vi "Auto_calibrate.vi"(3 "Mode":T4, 5 "Traverse line":T5 {"Row Duration (mins)" format="%#.1f"; "Row No" min=0; "Trace Gas Concentration (%)" min=0.0 format="%#.2f"; "Emission Rate (l/min)" format="%#.2f"; "Tunnel Speed" format="%#.2f"; "Start X" format="%#.2f"; "Start Y" format="%#.2f"; "Start Z" format="%#.2f"; "End X" format="%#.2f"; "End Y" format="%#.2f"; "End Z" format="%#.2f"; "Averaging time (min)" min=0.0 format="%#.2f"}) -> (0 "Error Messages":string, 1 "Status":T2, 2 "Traverse Out":T5 {"Row Duration (mins)" format="%#.1f"; "Row No" min=0; "Trace Gas Concentration (%)" min=0.0 format="%#.2f"; "Emission Rate (l/min)" format="%#.2f"; "Tunnel Speed" format="%#.2f"; "Start X" format="%#.2f"; "Start Y" format="%#.2f"; "Start Z" format="%#.2f"; "End X" format="%#.2f"; "End Y" format="%#.2f"; "End Z" format="%#.2f"; "Averaging time (min)" min=0.0 format="%#.2f"})   [LabVIEW 2012]
uses:
  Gen Trav/Traverse_cluster.ctl
  Gen Trav/Spacing.ctl
  Controls/Multi_run_mode.ctl
  Controls/User_Specific_mode.ctl
  Controls/Auto_Calib_Type.ctl
  Gen Trav/Multi_Run_Status.ctl
  Controls/Auto_Calib_Case.ctl
  File/Setup_Filetype.ctl
  Calibration/Calib_mode.ctl
  Controls/Setup.ctl
  Controls/Post_Process.ctl
  Controls/Save_Data.ctl
  Controls/App_Global.ctl
  Globals/Meas_global.vi
  Globals/Calib_global.vi
  Globals/Trav_pos_global.vi
  <vilib>/Analysis/baseanly.llb/Mean (DBL).vi
  Globals/Extra_Commands_Global.vi
  <vilib>/Analysis/NI_AALBase.lvlib
panel:
  out "Minimum St Dev":dbl[](array[numeric])
  out "Time FFID valve moved":dbl
  out "Wait factor":dbl
  out "Establishment time":string
  out "Orig Calib file string":string
  out "Concentrations":dbl[](array[numeric])
  out "FFID St Dev":dbl[][](array[numeric]) format="%.2f"
  in  "Clear Calib History":bool
  out "Coefficients":dbl[][](array[numeric]) format="%.2f"
  out "Currently in Case":T1
  out "Valve position":dbl format="%.2f"
  out "Currently On":i32
  out "Values":dbl[][](array[numeric]) format="%.2f"
  out "FF Indexes":i16[](array[numeric])
  out "Ch No's":i16[](array[numeric])
  out "No of Calib Points":i32
  out "Root Name":string[](array[string])
  out "Calibration varying":T3
  in  "stop":bool
  out "New Calib Filenames":path[](array[path])
  # "Specific Argument Options\n      Tunnel Speed;1;2;3;4\nOR  Traverse Position\nOR   Concentration"
  # "X           Y            Z"
  # "Start"
  # "End"
  # "X           Y            Z"
  # "Start"
  # "End"
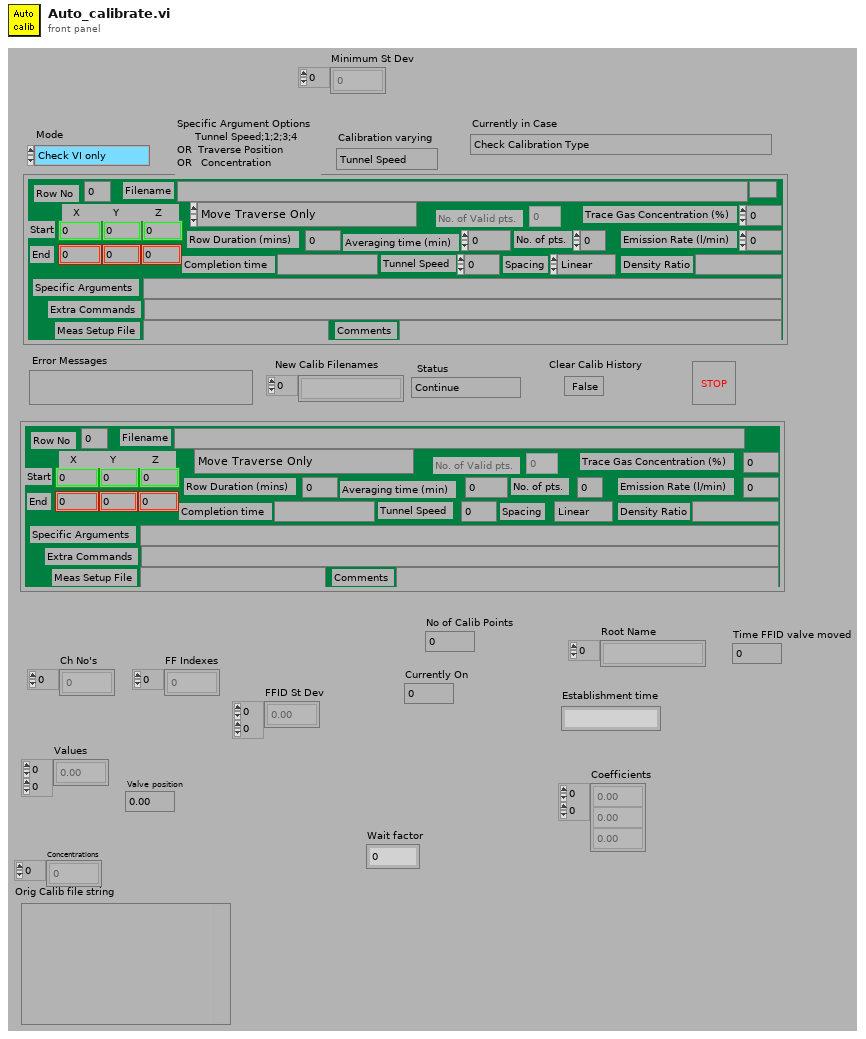
[diagram p1: front panel]
types:
  T1 = typedef "Auto_Calib_Case.ctl" = enum16{"Check Calibration Type", "Check if Original Calib file is Valid", "Get sampling rate etc. from meas setup file", "Setup Calibration Program", "Get Channel Numbers", "Check use latest selected on Mesurement setup files", "Create New Calib Filenames", "Setup Calibration Values in 2D array", "Create Measurement Setup File (Concentration Only)", "Are There Enough Calibration Points", "Set Measurement Conditions", "Measure Calibration Point", "Do Another Calibration Point?", "Skip Next Frame?", "Insert New calibration Filenames into Measurement Setup file", "Warn if FFID calibration is very non linear", "Warn if FFID variance is high", "Insert Bkgnd Variance into calib file", "Warn if FFID voltages are too low", "Warn if Current Calibration fit is poor", "Warn if Calibration Coefficients have significantly altered", "End"}
  T2 = typedef "Multi_Run_Status.ctl" = enum16{"Continue", "Jump to Next Point", "Jump to Next Row", "Jump To Fall Back", "Terminate Run"}
  T3 = typedef "Auto_Calib_Type.ctl" = enum16{"Tunnel Speed", "Traverse Position", "Concentration"}
  T4 = typedef "User_Specific_mode.ctl" = enum16{"Check VI only", "Run VI"}
  T5 = typedef "Traverse_cluster.ctl" = cluster{"Start X":dbl, "Start Y":dbl, "Start Z":dbl, "End X":dbl, "End Y":dbl, "End Z":dbl, "No. of pts.":i32, "Spacing":T6, "Filename":path, "Tunnel Speed":dbl, "Averaging time (min)":dbl, "Extra Commands":string, "Specific Arguments":string, "Emission Rate (l/min)":dbl, "Trace Gas Concentration (%)":dbl, "Density Ratio":string, "Comments":string, "Row No":i32, "Row Type Selector":T7, "Completion time":string, "Row Duration (mins)":dbl, "No. of Valid pts.":i32, "Meas Setup File":string}
  T6 = typedef "Spacing.ctl" = enum16{"Linear", "Log", "Gauss", "Specified", "N/A"}
  T7 = typedef "Multi_run_mode.ctl" = enum16{"Move Traverse Only", "Set Tunnel Speed Only", "Set Source Only", "Set Measurement Conditions", "Single Measurement", "Vertical Profile", "Lateral Profile", "Longitudinal Profile", "Explore Volume", "Multi-Axis Profile", "Auto Calibrate", "Meas Fast FID Bkgnd", "Check Beam Power", "Scanning Valve Measurement", "Run VI Named:", "Set ADAM Ch", "Wait (minutes)", "Send Message", "Synchronize With:", "Fall Back to this Row", "Turn Off Row Repeating", "Blank Row", "Traverse 3D Volume"}
  T8 = typedef "Setup_Filetype.ctl" = enum16{"Measurement Setups", "Calibration Setups", "General", "Results File Plotter Setups", "Speed Calib Tweaks"}
  T9 = typedef "Calib_mode.ctl" = enum16{"Show Setup", "Take a New Calibration Point", "Refit Curve", "Setup Front Panel"}
  T10 = typedef "Save_Data.ctl" = enum16{"Save No Data", "Save Data"}
  T11 = typedef "Post_Process.ctl" = enum16{"Take New Data", "Post Process Raw Data File"}
  T12 = typedef "Setup.ctl" = enum16{"Run Program", "Show Setup", "Save Current Setup", "Setup Front Panel"}
  T13 = typedef "App_Global.ctl" = enum16{"Read Global", "Write to Global", "Initialise Array"}
  T14 = typedef "Cal_Inst_type.ctl" = enum16{"Propeller anemometer", "Pressure Transducer", "Hot wire", "Cross wire velocity", "Cross wire angle", "Generic Linear", "Generic Polynomial", "Generic BackPoly", "Fast FID", "Thermocouple", "Cold wire", "Pulsed Wire"}
  T15 = typedef "Ref_Inst_type.ctl" = enum16{"Propellor anemometer", "Pressure Transducer", "Raw voltage", "Pitot-static tube", "Preston tube", "Generic Linear", "Generic Polynomial", "Thermocouple", "LDA", "Enter Value", "ADAM Channel"}
  T16 = cluster{"2nd Ref type":T15, "2nd inst present":bool}
  T17 = cluster{"high limit (10V)":sgl, "low limit (-10V)":sgl, "Ch No":i16, "Var name":string}[]
  T18 = cluster{"high limit (10V)":sgl, "low limit (-10V)":sgl, "Ch No":i16, "Var name":string}
  T19 = typedef "Inst_type.ctl" = enum16{"Propeller anemometer", "Raw voltage", "Pressure Transducer", "Pitot-static tube", "Preston tube", "Hot wire", "Cross wire 1", "Cross wire 2", "Generic Linear", "Generic Polynomial", "Generic BackPoly", "Fast FID", "Thermocouple", "Cold wire", "Pulsed Wire", "LDA Vel", "LDA Tran time", "LDA Arr time"}
  T20 = cluster{"high limit (10V)":sgl, "low limit (-10V)":sgl, "Ch No":i16, "Calib filename":path, "Inst type":T19, "Symbol":string, "Move channel":bool, "Use Latest":bool, "D":dbl, "Ch Name":string}[]
  T21 = typedef "Status_Cluster.ctl" = cluster{"Status":T2, "Error Type":string, "Error Description":string}
  T22 = typedef "Valco_valve_ph.ctl" = u16
  T23 = typedef "Time_Trace_Cluster.ctl" = cluster{"Weighting":dbl[], "Time (s)":dbl[], "Voltage":dbl[], "Eng Values":dbl[]}
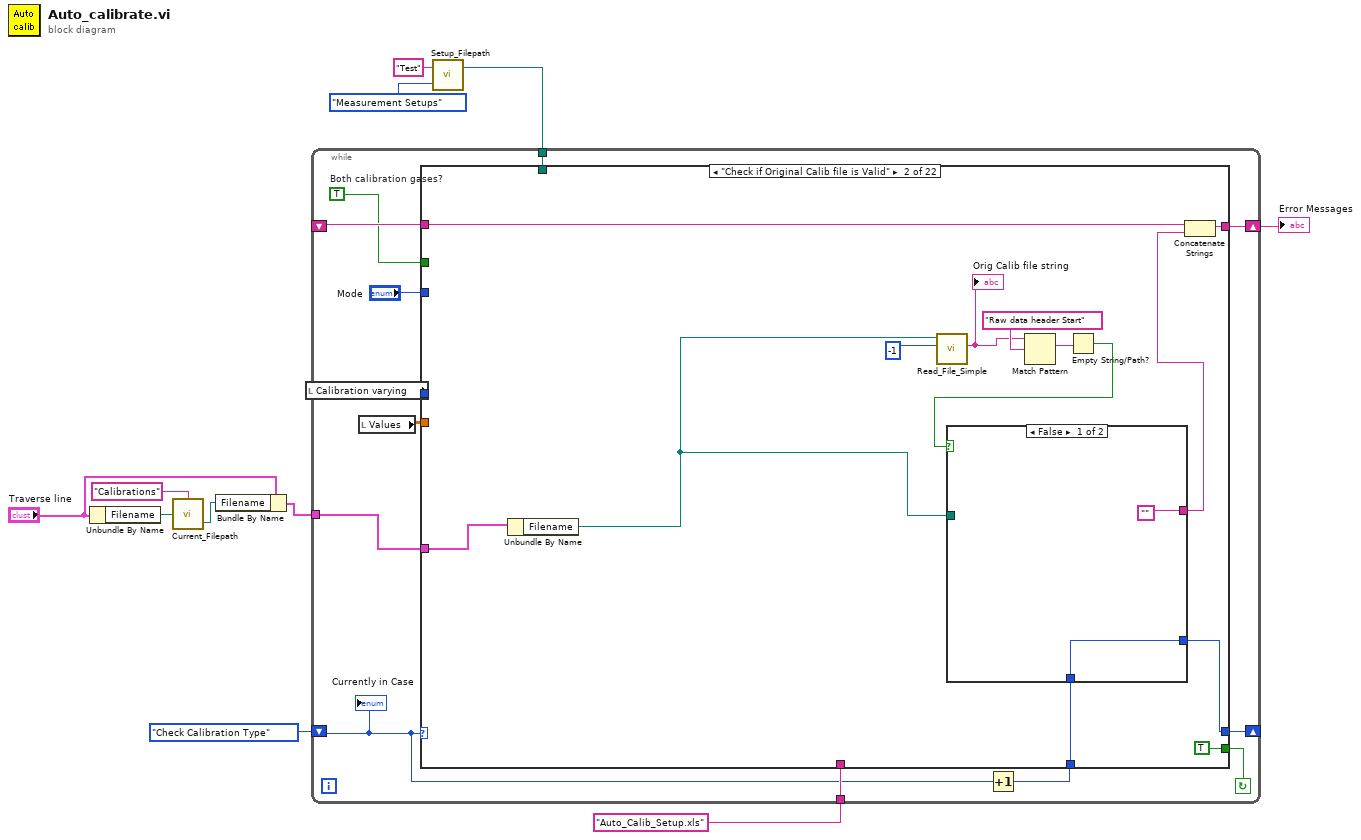
[diagram p0: block diagram]
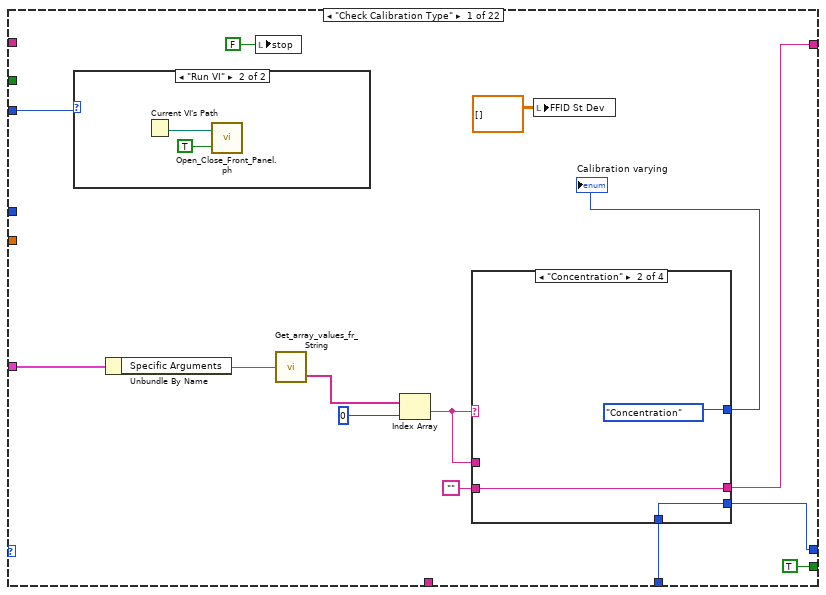
[diagram p2: hidden frame]
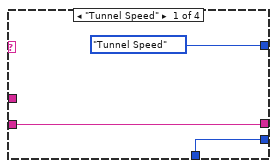
[diagram p4: hidden frame]
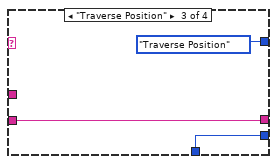
[diagram p5: hidden frame]
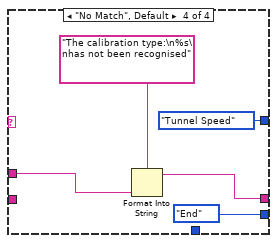
[diagram p6: hidden frame]
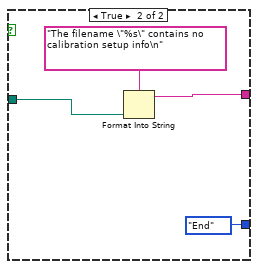
[diagram p7: hidden frame]
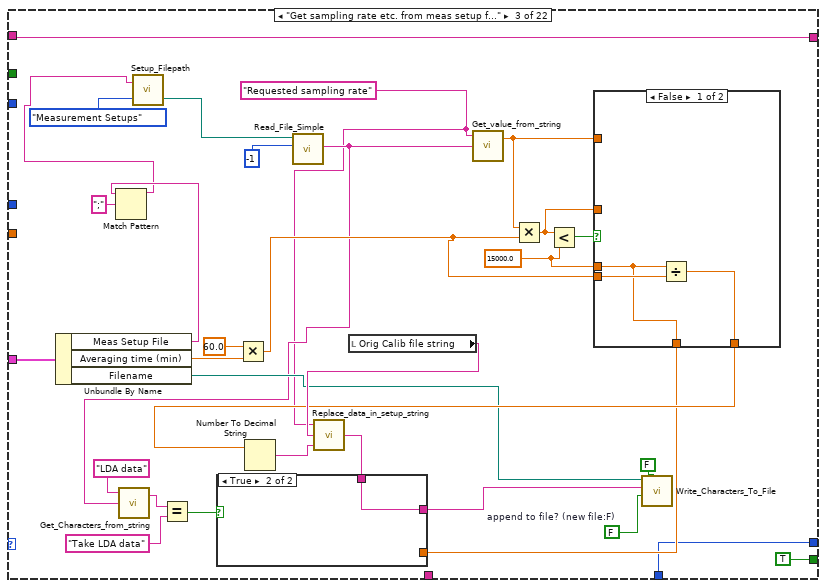
[diagram p8: hidden frame]
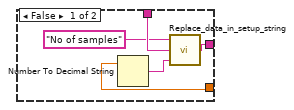
[diagram p9: hidden frame]
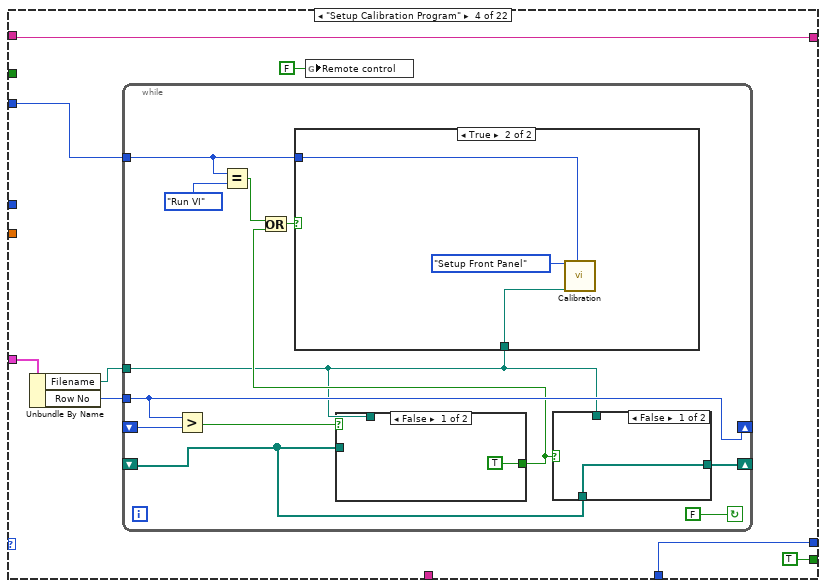
[diagram p11: hidden frame]
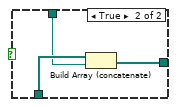
[diagram p12: hidden frame]
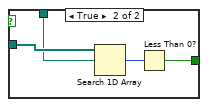
[diagram p14: hidden frame]
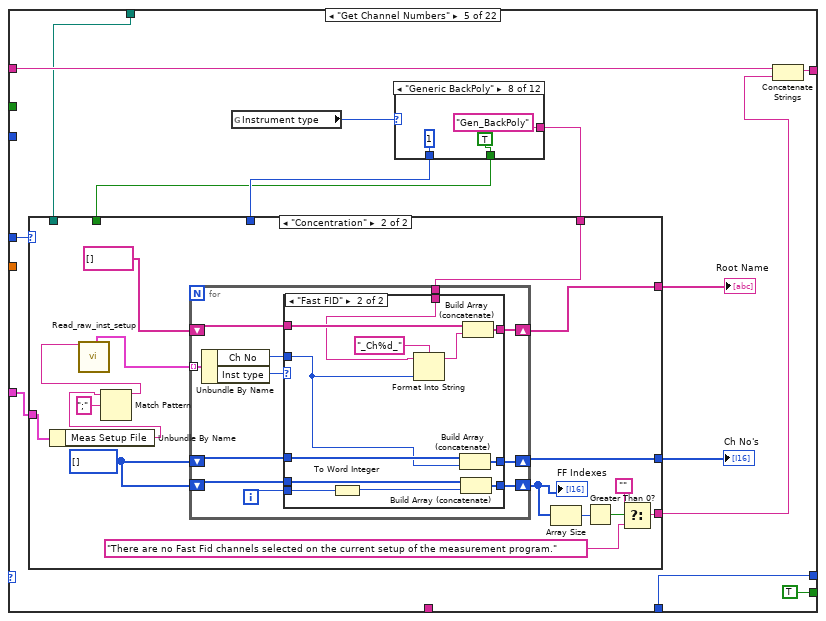
[diagram p15: hidden frame]
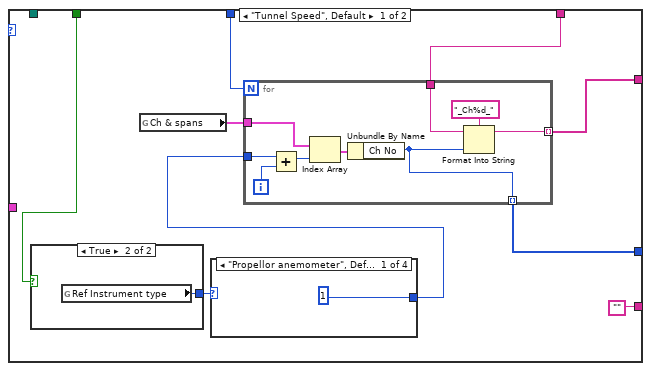
[diagram p16: hidden frame]
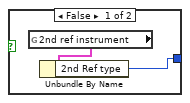
[diagram p17: hidden frame]
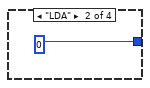
[diagram p18: hidden frame]
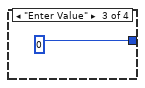
[diagram p19: hidden frame]
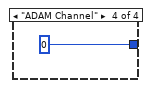
[diagram p20: hidden frame]
diagram:
  n1 = Unbundle By Name("Traverse line") -> ("Filename"=w4:path)
  n2 = call "Current_Filepath.vi"("Filename in"=w4, "Data Type"="Calibrations") -> ("Filename Out"=w3:path)  [unwired: 1 out]
  n3 = Bundle By Name(cluster="Traverse line", "Filename"=w3) -> (w1:T5)
  n4 = call "Setup_Filepath.vi"("Setup File Type"=Setup_Filetype."Measurement Setups", "Filename in"="Test") -> ("Directory"=w6:path)  [unwired: 1 out]
  n5 = while {
    shift-left: _ -> [w17]
    shift-right: [w18] -> w10
    shift-left: Auto_Calib_Case."Check Calibration Type" ("Currently in Case") -> [w16]
    shift-right: [w15] -> _
    tunnel: "Auto_Calib_Setup.xls" -> [w24]
    tunnel: w6 -> [w13]
    tunnel: w1 -> [w12]
    stop <- w21 continue-if-true
    w14 = TRUE  # Both calibration gases?
    n6 = local read "Calibration varying"() -> (w20:T3)
    n7 = local read "Values"() -> (w19:dbl[][])
    n8 = Increment(x=w16) -> (x+1=w22:T1)
    n9 = case shown="\"Check if Original Calib file is Valid\"" w16 {
      tunnel: w12 -> [w38 w67 w105 w120 w151 _ w319 w374 w407 _ w560 _ _ _ _ _ _ _ _ _ w977 w1008]
      tunnel: "Mode" -> [w29 _ _ w121 _ _ w326 _ w408 _ w555 _ w721 _ _ _ _ _ _ _ _ w1009]
      tunnel: w24 -> [_ _ _ _ _ _ _ _ w412 _ _ w632 _ _ _ _ _ _ _ _ _ _]
      tunnel: [w27 w57 w87 w123 w154 w270 w323 w365 w410 w523 w548 w631 w722 w748 w760 w779 w817 w882 w900 w956 w1000 w1013] -> w15
      tunnel: w22 -> [w28 w56 w87 w123 w154 w270 w323 w366 w410 w522 w542 w631 _ w747 w759 w779 w817 w882 w900 w956 w1000 w1013]
      tunnel: [TRUE TRUE TRUE TRUE TRUE TRUE TRUE TRUE w406 TRUE TRUE TRUE TRUE TRUE TRUE TRUE TRUE TRUE TRUE TRUE TRUE FALSE] -> w21
      tunnel: w20 -> [_ _ _ _ w158 _ w322 w372 _ _ w546 w633 w720 w746 w762 _ _ _ _ _ _ w1010]
      tunnel: w19 -> [_ _ _ _ _ _ _ _ w405 w532 w559 _ _ _ _ _ w824 _ w906 _ _ _]
      tunnel: [w31 w59 w85 w124 w155 w271 w336 w369 w411 w526 w543 w629 w719 w751 w766 w788 w831 w878 w907 w945 w993 w1012] -> w18
      tunnel: w17 -> [_ w61 w85 w124 w157 w271 w336 w368 w411 w527 w543 w629 w719 w751 w766 w788 w831 w878 w907 w945 w993 w1012]
      tunnel: w14 -> [_ _ _ _ _ _ _ w367 _ _ _ _ _ _ _ _ _ _ _ _ _ w1007]
      tunnel: w13 -> [_ _ _ _ w150 w273 _ _ w409 _ _ _ _ _ _ _ _ _ _ _ _ _]
      frame "Check Calibration Type" {
        n10 = case shown="\"Run VI\"" w29 {
          frame "Check VI only" {
          }
          frame "Run VI" {
            n11 = Current VI's Path() -> (path=w39:path)
            n12 = call "Open_Close_Front_Panel.ph.vi"("Front Panel Window:Open"=TRUE, "VI path"=w39) -> ()  [unwired: 2 out]
          }
        }
        n13 = Unbundle By Name(w38) -> ("Specific Arguments"=w37:string)
        n14 = local write "stop"(FALSE) -> ()
        n15 = call "Get_array_values_fr_String.vi"("String Value"=w37) -> ("String array"=w36:string[])  [unwired: 1 out]
        n16 = Index Array(array=w36, index=0 ("Index")) -> (element=w34:string)
        n17 = case shown="\"Concentration\"" w34 {
          tunnel: [Auto_Calib_Type."Tunnel Speed" ("Calibration varying") Auto_Calib_Type."Concentration" ("Calibration varying") Auto_Calib_Type."Traverse Position" ("Calibration varying") Auto_Calib_Type."Tunnel Speed" ("Calibration varying")] -> w32
          tunnel: w34 -> [_ _ _ w53]
          tunnel: [w42 w45 w48 w51] -> w31
          tunnel: "" -> [w42 w45 w48 _]
          tunnel: w28 -> [w41 w44 w47 _]
          tunnel: [w41 w44 w47 Auto_Calib_Case."End" ("Currently in Case")] -> w27
          frame "Tunnel Speed" {
          }
          frame "Concentration" {
            (unwired) ""
          }
          frame "Traverse Position" {
          }
          frame "No Match", Default {
            n18 = Format Into String(format string="The calibration type:\n%s\nhas not been recognised" ("Format String"), w53) -> (resulting string=w51:string)  [unwired: 2 in, 1 out]
          }
        }
        "Calibration varying" <- w32
        n19 = local write "FFID St Dev"(dbl[][] [] ("FFID Variance")) -> ()
      }
      frame "Check if Original Calib file is Valid" {
        n20 = Unbundle By Name(w67) -> ("Filename"=w55:path)
        n21 = call "Read_File_Simple.vi"("Filename"=w55, "number of characters (all:-1)"=-1) -> ("string"=w64:string)  [unwired: 1 in, 7 out]
        "Orig Calib file string" <- w64
        n22 = Match Pattern(string=w64, regular expression="Raw data header Start") -> (match substring=w63:string)  [unwired: 4 out]
        n23 = Empty String/Path?(string/path=w63) -> (empty?=w62:bool)
        n24 = case shown="False" w62 {
          tunnel: w55 -> [_ w73]
          tunnel: ["" w71] -> w60
          tunnel: [w68 Auto_Calib_Case."End" ("Currently in Case")] -> w57
          tunnel: w56 -> [w68 _]
          frame False {
          }
          frame True {
            n25 = Format Into String(format string="The filename \"%s\" contains no calibration setup info\n" ("Format String"), w73) -> (resulting string=w71:string)  [unwired: 2 in, 1 out]
          }
        }
        n26 = Concatenate Strings(w61, w60) -> (w59:string)
      }
      frame "Get sampling rate etc. from meas setup file" {
        w88 = FALSE  # append to file? (new file:F)
        w77 = "Requested sampling rate"
        w95 = 15000.0 ("y")
        n27 = Unbundle By Name(w105) -> ("Meas Setup File"=w83:string, "Averaging time (min)"=w103:dbl, "Filename"=w90:path)
        n28 = Match Pattern(string=w83, regular expression=";") -> (before substring=w75:string)  [unwired: 4 out]
        n29 = call "Setup_Filepath.vi"("Setup File Type"=Setup_Filetype."Measurement Setups", "Filename in"=w75) -> ("Filename Out"=w74:path)  [unwired: 1 out]
        n30 = Multiply(x=60.0, y=w103) -> (x*y=w94:dbl)
        n31 = call "Read_File_Simple.vi"("Filename"=w74, "number of characters (all:-1)"=-1) -> ("string"=w82:string)  [unwired: 1 in, 7 out]
        n32 = call "Get_Characters_from_string.vi"("Input string"=w82, "Variable name"="LDA data") -> ("Value"=w80:string)  [unwired: 1 in, 1 out]
        n33 = Equal?(x=w80, y="Take LDA data") -> (x = y?=w78:bool)
        n34 = local read "Orig Calib file string"() -> (w99:string)
        n35 = call "Get_value_from_string.vi"("Input string"=w82, "Variable name"=w77) -> ("Value"=w98:dbl)  [unwired: 1 in, 1 out]
        n36 = Multiply(x=w98, y=w94) -> (x*y=w93:dbl)
        n37 = Less?(x=w93, y=w95) -> (x < y?=w101:bool)
        n38 = case shown="False" w101 {
          tunnel: w98 -> [_ w116]
          tunnel: [w113 w116] -> w97
          tunnel: w95 -> [w112 _]
          tunnel: w94 -> [w114 _]
          tunnel: [w112 w115] -> w91
          tunnel: w93 -> [_ w115]
          frame False {
            n39 = Divide(x=w112, y=w114) -> (x/y=w113:dbl)
          }
          frame True {
          }
        }
        n40 = Number To Decimal String(number=w97) -> (decimal integer string=w96:string)  [unwired: 1 out]
        n41 = call "Replace_data_in_setup_string.vi"("New data string"=w96, "Input string"=w99, "Variable name"=w77) -> ("Appended string"=w92:string)
        n42 = case shown="True" w78 {
          tunnel: w92 -> [w110 w111]
          tunnel: w91 -> [w107 _]
          tunnel: [w106 w111] -> w89
          frame False {
            n43 = Number To Decimal String(number=w107) -> (decimal integer string=w108:string)  [unwired: 1 out]
            n44 = call "Replace_data_in_setup_string.vi"("New data string"=w108, "Input string"=w110, "Variable name"="No of samples") -> ("Appended string"=w106:string)
          }
          frame True {
          }
        }
        n45 = call "Write_Characters_To_File.vi"("file path (dialog if empty)"=w90, "advisory dialog? (display:T)"=FALSE, "character string"=w89, "append to file? (new file:F)"=w88) -> ()  [unwired: 1 in, 4 out]
      }
      frame "Setup Calibration Program" {
        n46 = Unbundle By Name(w120) -> ("Filename"=w117:path, "Row No"=w119:i32)
        n47 = while {
          shift-left: _ -> [w128]
          shift-right: [w127] -> _
          tunnel: w119 -> [w135]
          shift-left: _ -> [w136]
          shift-right: [w135] -> _
          tunnel: w121 -> [w133]
          tunnel: w117 -> [w125]
          stop <- FALSE continue-if-true
          n48 = Greater?(x=w135, y=w136) -> (0:w134:bool)
          n49 = Equal?(x=w133, y=User_Specific_mode."Run VI" ("Mode")) -> (x = y?=w131:bool)
          n50 = case shown="False" w134 {
            tunnel: w128 -> [_ w148]
            tunnel: w125 -> [_ w147]
            tunnel: [TRUE w145] -> w129
            frame False {
            }
            frame True {
              n51 = Search 1D Array(1D array=w148, element=w147) -> (index of element=w146:i32)  [unwired: 1 out]
              n52 = Less Than 0?(x=w146) -> (x < 0?=w145:bool)
            }
          }
          n53 = Or(x=w131, y=w129) -> (x .or. y?=w130:bool)
          n54 = case shown="True" w130 {
            tunnel: w133 -> [_ w143]
            tunnel: w125 -> [_ w142]
            frame False {
            }
            frame True {
              n55 = call "Calibration.vi"("Mode"=Calib_mode."Setup Front Panel", "Calib file"=w142, "Simulate/Run"=w143) -> ()  [unwired: 17 out]
            }
          }
          n56 = case shown="False" w129 {
            tunnel: w128 -> [w137 w140]
            tunnel: w125 -> [_ w139]
            tunnel: [w137 w138] -> w127
            frame False {
            }
            frame True {
              n57 = Build Array (concatenate)(w140, w139) -> (w138:path[])
            }
          }
        }
        n58 = global write "Meas_global.vi" "Remote control"(FALSE ("Remote control")) -> ()
      }
      frame "Get Channel Numbers" {
        n59 = global read "Calib_global.vi" "Instrument type"() -> (w162:T14)
        n60 = case shown="\"Generic BackPoly\"" w162 {
          tunnel: ["Prop" "Mano" "HW" "XW" "XW" "Gen_Lin" "Gen_Poly" "Gen_BackPoly" "FF" "Therm" "CW" "PWA"] -> w161
          tunnel: [1 1 1 2 2 1 1 1 1 1 1 1] -> w152
          tunnel: [TRUE TRUE TRUE TRUE FALSE TRUE TRUE TRUE TRUE TRUE TRUE TRUE] -> w149
          frame "Propeller anemometer" {
          }
          frame "Pressure Transducer" {
          }
          frame "Hot wire" {
          }
          frame "Cross wire velocity" {
          }
          frame "Cross wire angle" {
          }
          frame "Generic Linear" {
          }
          frame "Generic Polynomial" {
          }
          frame "Generic BackPoly" {
          }
          frame "Fast FID" {
          }
          frame "Thermocouple" {
          }
          frame "Cold wire" {
          }
          frame "Pulsed Wire" {
          }
        }
        n61 = case shown="\"Concentration\"" w158 {
          tunnel: w161 -> [w169 w203]
          tunnel: [w165 w202] -> w160
          tunnel: [w166 w200] -> w159
          tunnel: ["" w193] -> w156
          tunnel: w152 -> [w167 _]
          tunnel: w151 -> [_ w192]
          tunnel: w150 -> [_ _]
          tunnel: w149 -> [w163 _]
          frame "Tunnel Speed", Default {
            n62 = case shown="True" w163 {
              tunnel: [w172 w174] -> w171
              frame False {
                n63 = global read "Calib_global.vi" "2nd ref instrument"() -> (w173:T16)
                n64 = Unbundle By Name(w173) -> ("2nd Ref type"=w172:T15)
              }
              frame True {
                n65 = global read "Calib_global.vi" "Ref Instrument type"() -> (w174:T15)
              }
            }
            n66 = global read "Calib_global.vi" "Ch & spans"() -> (w168:T17)
            n67 = case shown="\"Propellor anemometer\", Default" w171 {
              tunnel: [1 i16 0 0 0] -> w164
              frame "Propellor anemometer", Default {
              }
              frame "LDA" {
              }
              frame "Enter Value" {
              }
              frame "ADAM Channel" {
              }
            }
            n68 = for {
              N: w167 -> [_]
              tunnel: [w181] -> w166 mode=indexing
              tunnel: w169 -> [w180]
              tunnel: w168 -> [w179]
              tunnel: [w178] -> w165 mode=indexing
              tunnel: w164 -> [w176]
              i -> [w177]
              n69 = Add(x=w176, y=w177) -> (x+y=w175:i32)
              n70 = Index Array(array=w179, index=w175) -> (element=w183:T18)
              n71 = Unbundle By Name(w183) -> ("Ch No"=w181:i16)
              n72 = Format Into String(format string="_Ch%d_" ("Format String"), initial string=w180, w181) -> (resulting string=w178:string)  [unwired: 1 in, 1 out]
            }
          }
          frame "Concentration" {
            w199 = i16[] []
            n73 = Unbundle By Name(w192) -> ("Meas Setup File"=w189:string)
            n74 = Match Pattern(string=w189, regular expression=";") -> (before substring=w188:string)  [unwired: 4 out]
            n75 = call "Read_raw_inst_setup.vi"("Setup file"=w188) -> ("Ch & spans choices"=w191:T20)  [unwired: 18 out]
            n76 = for {
              tunnel: w191 -> [w214] mode=indexing
              tunnel: w203 -> [w213]
              shift-right: [w209] -> w202
              shift-left: string[] [] -> [w210]
              shift-right: [w207] -> w200
              shift-left: w199 -> [w208]
              shift-right: [w206] -> w198
              shift-left: w199 -> [w205]
              i -> [w204]
              n77 = Unbundle By Name(w214) -> ("Ch No"=w212:i16, "Inst type"=w211:T19)
              n78 = case shown="\"Fast FID\"" w211 {
                tunnel: w213 -> [_ w219]
                tunnel: w212 -> [_ w221]
                tunnel: w210 -> [w217 w229]
                tunnel: [w217 w228] -> w209
                tunnel: w208 -> [w216 w227]
                tunnel: [w216 w226] -> w207
                tunnel: w205 -> [w215 w224]
                tunnel: [w215 w225] -> w206
                tunnel: w204 -> [_ w223]
                frame "Generic Linear", Default {
                }
                frame "Fast FID" {
                  n79 = To Word Integer(number=w223) -> (16bit integer=w222:i16)
                  n80 = Format Into String(format string="_Ch%d_", initial string=w219, w221) -> (resulting string=w218:string)  [unwired: 1 in, 1 out]
                  n81 = Build Array (concatenate)(w227, w221) -> (w226:i16[])
                  n82 = Build Array (concatenate)(w224, w222) -> (w225:i16[])
                  n83 = Build Array (concatenate)(w229, w218) -> (w228:string[])
                }
              }
            }
            "FF Indexes" <- w198
            n84 = Array Size(array=w198) -> (size(s)=w197:i32)
            n85 = Greater Than 0?(x=w197) -> (x > 0?=w196:bool)
            n86 = Select(t="", s=w196, f="There are no Fast Fid channels selected on the current setup of the measurement program.") -> (s? t:f=w193:string)
          }
        }
        "Root Name" <- w160
        "Ch No's" <- w159
        n87 = Concatenate Strings(w157, w156) -> (w155:string)
      }
      frame "Check use latest selected on Mesurement setup files" {
        n88 = global read "Trav_pos_global.vi" "Measurement setup files"() -> (w266:string[])
        n89 = local read "Ch No's"() -> (w272:i16[])
        n90 = Build Array (concatenate)(w266, "Current_Setup.xls") -> (w267:string[])
        n91 = for {
          tunnel: w273 -> [w276]
          tunnel: w267 -> [w275] mode=indexing
          tunnel: w272 -> [w274]
          n92 = stacked-sequence {
            seq-local: [w277 _ _] -> [_ w283 w311]
            seq-local: [_ w281 _] -> [_ _ w309]
            tunnel: w276 -> [w280 _ w308]
            tunnel: w275 -> [w279 _ w307]
            tunnel: w274 -> [_ w282 _]
            frame #0 {
              n93 = Build Path(base path=w280, name or relative path=w279) -> (appended path=w278:path)
              n94 = call "Read_File_Simple.vi"("Filename"=w278) -> ("string"=w277:string)  [unwired: 2 in, 7 out]
            }
            frame #1 {
              n95 = while {
                shift-right: [w288] -> w281
                shift-left: w283 -> [w289]
                tunnel: w282 -> [w292]
                i -> [w296]
                stop <- w285 continue-if-true
                n96 = Increment(x=w296) -> (x+1=w290:i32)
                n97 = Format Into String(format string="An ch %d Ch No", w290) -> (resulting string=w295:string)  [unwired: 2 in, 1 out]
                n98 = call "Get_value_from_string.vi"("Input string"=w289, "Variable name"=w295) -> ("Status"=w294:enum16{"Char in string", "Char not in string"}, "Value"=w293:dbl)  [unwired: 1 in]
                n99 = To Long Integer(number=w293) -> (32bit integer=w291:i32)
                n100 = Search 1D Array(1D array=w292, element=w291) -> (index of element=w287:i32)  [unwired: 1 in]
                n101 = Greater Or Equal To 0?(x=w287) -> (x >= 0?=w286:bool)
                n102 = case shown="\"Char in string\"" w294 {
                  tunnel: [TRUE FALSE] -> w285
                  frame "Char in string" {
                  }
                  frame "Char not in string" {
                  }
                }
                n103 = And(x=w286, y=w285) -> (x .and. y?=w284:bool)
                n104 = case shown="True" w284 {
                  tunnel: w290 -> [w300 _]
                  tunnel: w289 -> [w299 w304]
                  tunnel: [w298 w304] -> w288
                  frame True {
                    n105 = Format Into String(format string="An ch %d Use latest Calib", w300) -> (resulting string=w302:string)  [unwired: 2 in, 1 out]
                    n106 = call "Replace_data_in_setup_string.vi"("New data string"="TRUE" ("Replace with"), "Input string"=w299, "Variable name"=w302) -> ("Appended string"=w298:string)
                  }
                  frame False {
                  }
                }
              }
            }
            frame #2 {
              n107 = Equal?(x=w311, y=w309) -> (x = y?=w310:bool)
              n108 = case shown="True" w310 {
                tunnel: w308 -> [w314 _]
                tunnel: w309 -> [w317 _]
                tunnel: w307 -> [w313 _]
                frame False {
                  w316 = FALSE  # append to file? (new file:F)
                  n109 = Build Path(base path=w314, name or relative path=w313) -> (appended path=w312:path)
                  n110 = call "Write_Characters_To_File.vi"("file path (dialog if empty)"=w312, "advisory dialog? (display:T)"=FALSE, "character string"=w317, "append to file? (new file:F)"=w316) -> ()  [unwired: 1 in, 4 out]
                }
                frame True {
                }
              }
            }
          }
        }
      }
      frame "Create New Calib Filenames" {
        n111 = Unbundle By Name(w319) -> ("Filename"=w318:path)
        n112 = Get Date/Time String(date format (0)=enum16{"short", "long", "abbreviated"}."short") -> (date string=w330:string)  [unwired: 3 out]
        n113 = Strip Path(path=w318) -> (stripped path=w325:path)  [unwired: 1 out]
        n114 = local read "Root Name"() -> (w321:string[])
        n115 = case shown="\"Tunnel Speed\", Default" w322 {
          tunnel: w321 -> [_ w341]
          tunnel: [1 w340] -> w320
          frame "Tunnel Speed", Default {
          }
          frame "Concentration" {
            n116 = Array Size(array=w341) -> (size(s)=w340:i32)
          }
        }
        n117 = call "Replace_Character.vi"("Replace with"="-", "Input String"=w330, "Search For"="/") -> ("Output string"=w327:string)  [unwired: 1 out]
        n118 = List Folder(path=w325) -> (filenames=w338:string[])  [unwired: 1 in, 5 out]
        n119 = To Upper Case(1:w338) -> (0:w337:string[])
        n120 = for {
          N: w320 -> [_]
          tunnel: w321 -> [w344] mode=indexing
          tunnel: w337 -> [w348]
          tunnel: w325 -> [w347]
          tunnel: [w343] -> w334 mode=indexing
          tunnel: w327 -> [w345]
          tunnel: w326 -> [w342]
          n121 = while {
            tunnel: w344 -> [w355]
            tunnel: w345 -> [w356]
            tunnel: [w351] -> w346
            tunnel: w348 -> [w358]
            i -> [w360]
            stop <- w362 continue-if-true
            n122 = Increment(x=w360) -> (x+1=w357:i32)
            n123 = Format Into String(format string="%s_%d.xls" ("Format String"), initial string=w355, w356, w357) -> (resulting string=w352:string)  [unwired: 1 in, 1 out]
            n124 = call "Replace_Character.vi"("Replace with"="_", "Input String"=w352, "Search For"=" ") -> ("Output string"=w351:string)  [unwired: 1 out]
            n125 = To Upper Case(1:w351) -> (0:w361:string)
            n126 = Search 1D Array(1D array=w358, element=w361) -> (index of element=w363:i32)  [unwired: 1 out]
            n127 = Not Equal?(x=w363, y=-1) -> (x != y?=w362:bool)
          }
          n128 = Build Path(base path=w347, name or relative path=w346) -> (appended path=w343:path)
          n129 = case shown="\"Run VI\"" w342 {
            tunnel: w343 -> [_ w349]
            frame "Check VI only" {
            }
            frame "Run VI" {
              n130 = call "Calibration.vi"("Mode"=Calib_mode."Setup Front Panel", "Calib file"=w349) -> ()  [unwired: 1 in, 17 out]
            }
          }
        }
        "New Calib Filenames" <- w334
        n131 = Index Array(array=w334, index=0 ("Index")) -> (element=w332:path)
        n132 = global write "Meas_global.vi" "Results file"(w332) -> ()
        "Establishment time" <- "!Establish Exp Conditions (s) = 15" ("Message")
      }
      frame "Setup Calibration Values in 2D array" {
        n133 = case shown="\"Tunnel Speed\"" w372 {
          tunnel: [w383 w389 w404] -> w371
          tunnel: w374 -> [w378 _ w403]
          tunnel: ["" "" w402] -> w370
          tunnel: w367 -> [_ w387 _]
          tunnel: w366 -> [w377 w386 w401]
          tunnel: [w376 w386 w400] -> w365
          frame "Tunnel Speed" {
            n134 = Unbundle By Name(w378) -> ("Specific Arguments"=w381:string)
            n135 = call "Get_array_values_fr_String.vi"("String Value"=w381) -> ("Numeric Array"=w379:dbl[])  [unwired: 1 out]
            n136 = Array Subset(array=w379, index=1 ("Array Index")) -> (w375:dbl[])  [unwired: 1 in]
            n137 = for {
              tunnel: w375 -> [w385] mode=indexing
              tunnel: [w384] -> w383 mode=indexing
              n138 = Build Array(w385) -> (w384:dbl[])
            }
            n139 = Increment(x=w377) -> (x+1=w376:T1)
          }
          frame "Concentration" {
            n140 = case shown="True" w387 {
              tunnel: [w391 w395] -> w390
              frame True {
                n141 = Build Array(3.0, 2.0, 1.0) -> (w391:dbl[])
              }
              frame False {
                n142 = Build Array(1.0, 3.0) -> (w395:dbl[])
              }
            }
            n143 = for {
              tunnel: w390 -> [w399] mode=indexing
              tunnel: [w398] -> w389 mode=indexing
              n144 = Build Array(w399) -> (w398:dbl[])
            }
          }
          frame "Traverse Position" {
            n145 = call "Create_Pos_array.vi"("Traverse line"=w403) -> ("Error Messages"=w402:string, "Array of Positions"=w404:dbl[][])  [unwired: 5 in, 2 out]
            n146 = Increment(x=w401) -> (x+1=w400:T1)
          }
        }
        "Values" <- w371
        n147 = Concatenate Strings(w368, w370) -> (w369:string)
      }
      frame "Create Measurement Setup File (Concentration Only)" {
        n148 = stacked-sequence {
          seq-local: [w423 _ _ _ _ _] -> [_ w442 _ _ _ _]
          seq-local: [_ w440 _ _ _ _] -> [_ _ w463 _ _ _]
          tunnel: w409 -> [w414 _ w464 _ _ _]
          tunnel: w412 -> [_ _ w465 _ _ _]
          tunnel: w408 -> [_ _ _ w471 w490 w507]
          tunnel: w407 -> [w420 _ _ _ w491 _]
          tunnel: [_ _ _ _ w489 _] -> w406
          tunnel: w405 -> [_ _ _ w474 _ _]
          frame #0 {
            w427 = TRUE  # Show Dialog?
            n149 = Unbundle By Name(w420) -> ("Meas Setup File"=w421:string)
            n150 = Match Pattern(string=w421, regular expression=";") -> (before substring=w419:string)  [unwired: 4 out]
            n151 = Build Path(base path=w414, name or relative path=w419) -> (appended path=w428:path)
            n152 = Format Into String(format string="Meas Setup File   %s", w414) -> (resulting string=w413:string)  [unwired: 2 in, 1 out]
            n153 = call "Read_spec_No_of_Characters.vi"("Filename"=w428) -> ("character string"=w429:string)  [unwired: 1 out]
            n154 = call "Get_string_subset.vi"("String Name"=w413, "Show Dialog?"=w427, "String to split"=w429, "File Label"="Raw data header") -> ("Output string"=w416:string)  [unwired: 1 out]
            n155 = call "Get_value_from_string.vi"("Input string"=w416, "Variable name"="No of analogue inst") -> ("Value"=w417:dbl)  [unwired: 1 in, 1 out]
            n156 = for {
              N: w417 -> [_]
              shift-right: [w431] -> w426
              shift-left: w416 -> [w433]
              i -> [w437]
              n157 = Increment(x=w437) -> (x+1=w436:i32)
              n158 = Number To Decimal String(number=w436) -> (decimal integer string=w439:string)  [unwired: 1 out]
              n159 = Concatenate Strings("An ch ", w439, " Inst type") -> (w434:string)
              n160 = call "Replace_data_in_setup_string.vi"("New data string"="Raw voltage", "Input string"=w433, "Variable name"=w434) -> ("Appended string"=w431:string)
            }
            n161 = call "Replace_data_in_setup_string.vi"("New data string"="No LDA data", "Input string"=w426, "Variable name"="LDA data" ("Label for characters")) -> ("Appended string"=w423:string)
          }
          frame #1 {
            n162 = global read "Calib_global.vi" "New Setup String"() -> (w443:string)
            n163 = for {
              N: 4 -> [_]
              shift-right: [w448] -> w440
              shift-left: w442 -> [w449]
              tunnel: w443 -> [w445]
              i -> [w447]
              n164 = case shown="3" w447 {
                tunnel: [w452 w455 w458 "No of blocks"] -> w446
                tunnel: w445 -> [w451 w454 w457 _]
                tunnel: [w450 w453 w456 "1" ("Value")] -> w444
                frame 0, Default {
                  w452 = "No of samples"
                  n165 = call "Get_Characters_from_string.vi"("Input string"=w451, "Variable name"=w452) -> ("Value"=w450:string)  [unwired: 1 in, 1 out]
                }
                frame 2 {
                  w455 = "Actual sampling rate"
                  n166 = call "Get_Characters_from_string.vi"("Input string"=w454, "Variable name"=w455) -> ("Value"=w453:string)  [unwired: 1 in, 1 out]
                }
                frame 3 {
                  w458 = "Board type"
                  n167 = call "Get_Characters_from_string.vi"("Input string"=w457, "Variable name"=w458) -> ("Value"=w456:string)  [unwired: 1 in, 1 out]
                }
                frame 1 {
                }
              }
              n168 = call "Replace_data_in_setup_string.vi"("New data string"=w444, "Input string"=w449, "Variable name"=w446) -> ("Appended string"=w448:string)
            }
          }
          frame #2 {
            w469 = FALSE  # advisory dialog? (display:T)
            w470 = FALSE  # append to file? (new file:F)
            n169 = call "Remove_Plug_Ins_etc.vi"("Input String"=w463) -> ("Output string"=w462:string)
            n170 = call "Add_label_to_string.vi"("String to write"=w462, "File Label"="Raw data header") -> ("Output string"=w466:string)
            n171 = Build Path(base path=w464, name or relative path=w465) -> (appended path=w461:path)
            n172 = call "Add_length_to_string.vi"("String in"=w466) -> ("String out"=w468:string)
            n173 = call "Write_Characters_To_File.vi"("file path (dialog if empty)"=w461, "advisory dialog? (display:T)"=w469, "character string"=w468, "append to file? (new file:F)"=w470) -> ()  [unwired: 1 in, 4 out]
          }
          frame #3 {
            w473 = 0 ("Index")
            w478 = 0.0 ("Input Element")
            n174 = Index Array(array=w474, index (row)=w473, index (col)=w473) -> (element=w472:dbl)
            n175 = case shown="\"Run VI\"" w471 {
              tunnel: w472 -> [_ w481]
              frame "Check VI only" {
              }
              frame "Run VI" {
                n176 = flat-sequence {
                  tunnel: w481 -> [w482]
                  frame #0 {
                    n177 = call "Fast_FID_Valve_Control.vi"("Requested Position"=w482) -> ()  [unwired: 7 out]
                  }
                  frame #1 {
                    n178 = Get Date/Time In Seconds() -> (seconds since 1Jan1904=w484:timestamp)
                    n179 = To Double Precision Float(number=w484) -> (double precision float=→"Time FFID valve moved":dbl)
                  }
                }
              }
            }
            n180 = Build Array("GMU:Calibration:Gas 1", "GMU:Calibration:Gas 2") -> (w480:string[])
            n181 = call "Get_Current_Scan_client.vi"("ADAM Ch Names"=w480) -> ("Numerical Values"=w479:dbl[])  [unwired: 3 out]
            n182 = Build Array (concatenate)(w478, w478, w479, w478) -> (→"Concentrations":dbl[])
          }
          frame #4 {
            w488 = dbl[] [30.0, 15.0, 0.0] ("appended array")
            n183 = Unbundle By Name(w491) -> ("Start Z"=w485:dbl)
            n184 = Array Size(array=w488) -> (size(s)=w487:i32)
            n185 = Decrement(x=w487) -> (x-1=w486:i32)
            n186 = while {
              tunnel: w490 -> [w500]
              tunnel: w491 -> [w504]
              tunnel: w488 -> [w503] mode=indexing
              tunnel: w485 -> [w501]
              tunnel: w486 -> [w496]
              tunnel: [w492] -> w489
              i -> [w497]
              stop <- w493 continue-if-true
              n187 = Add(x=w501, y=w503) -> (x+y=w502:dbl)
              n188 = Less?(x=w497, y=w496) -> (x < y?=w494:bool)
              n189 = Bundle By Name(cluster=w504, "Start Z"=w502) -> (w505:T5)
              n190 = call "Set_Traverse_Position.vi"("Simulate/Run"=w500, "Currently on Point"=1, "Traverse line"=w505) -> ("Status Cluster"=w495:T21)  [unwired: 2 out]
              n191 = Unbundle By Name(w495) -> ("Status"=w498:T2)
              n192 = call "Prog_Status_Handler.vi"("Status Cluster"=w495, "Simulate/Run"=w500) -> ()  [unwired: 2 out]
              n193 = local write "Status"(w498) -> ()
              n194 = Equal?(x=w498, y=Multi_Run_Status."Continue" ("Status")) -> (x = y?=w492:bool)
              n195 = And(x=w492, y=w494) -> (x .and. y?=w493:bool)
            }
          }
          frame #5 {
            n196 = case shown="\"Run VI\"" w507 {
              frame "Check VI only", Default {
              }
              frame "Run VI" {
                n197 = while {
                  shift-right: [w519] -> _
                  shift-left: _ -> [w520]
                  tunnel: [w518] -> w513
                  stop <- TRUE stop-if-true
                  n198 = Get Date/Time In Seconds() -> (seconds since 1Jan1904=w519:timestamp)
                  n199 = Subtract(x=w519, y=w520) -> (x-y=w518:dbl)
                }
                n200 = Divide(x=w513, y=3600.0) -> (x/y=w512:dbl)
                n201 = Multiply(x=w512, y=0.2) -> (x*y=w510:dbl)
                n202 = Add(x=w510, y=0.8) -> (x+y=w508:dbl)
                n203 = In Range and Coerce(upper limit=2.0, x=w508, lower limit=1.0) -> (coerced(x)=→"Wait factor":dbl)  [unwired: 1 out]
              }
            }
          }
        }
      }
      frame "Are There Enough Calibration Points" {
        n204 = Array Size(array=w532) -> (size(s)=w533:i32[])
        n205 = Index Array(array=w533, index=0 ("Index")) -> (element=w528:i32)
        "No of Calib Points" <- w528
        n206 = Greater?(x=w528, y=1) -> (0:w529:bool)
        n207 = case shown="False" w529 {
          tunnel: ["Less than two calibration points have been specified\n" ""] -> w525
          tunnel: [Auto_Calib_Case."End" ("Currently in Case") w537] -> w523
          tunnel: w522 -> [_ w537]
          frame False {
          }
          frame True {
          }
        }
        n208 = Concatenate Strings(w527, w525) -> (w526:string)
        "Currently On" <- 1 ("Currently On")
      }
      frame "Set Measurement Conditions" {
        n209 = local read "Currently On"() -> (w547:i32)
        n210 = Decrement(x=w547) -> (x-1=w558:i32)
        n211 = Index Array(array=w559, index (row)=w558) -> (element=w557:dbl[])  [unwired: 1 in]
        n212 = case shown="\"Concentration\"" w546 {
          tunnel: w557 -> [w575 w592 w609]
          tunnel: w555 -> [_ _ w607]
          tunnel: w560 -> [w573 w588 w598]
          tunnel: [w574 w587 w596] -> w541
          tunnel: w547 -> [w569 _ w599]
          tunnel: [w572 w586 w603] -> w539
          frame "Tunnel Speed" {
            n213 = Index Array(array=w575, index=0 ("Index")) -> (element=w562:dbl)
            n214 = while {
              shift-right: [w583] -> w564
              shift-left: _ -> [w582]
              tunnel: w562 -> [w585]
              tunnel: [w583] -> w571
              tunnel: [w582] -> w570
              stop <- FALSE continue-if-true
              n215 = Greater Than 0?(x=w585) -> (x > 0?=w583:bool)
            }
            n216 = Exclusive Or(1:w570, 2:w571) -> (0:w567:bool)
            n217 = Greater?(x=w569, y=1) -> (0:w566:bool)
            n218 = And(x=w567, y=w566) -> (x .and. y?=w565:bool)
            n219 = case shown="False" w564 {
              tunnel: [w577 w579] -> w563
              tunnel: w562 -> [w578 w579]
              frame False {
                n220 = Negate(x=w578) -> (-x=w577:dbl)
              }
              frame True {
              }
            }
            n221 = case shown="True" w565 {
              frame False {
              }
              frame True {
                n222 = call "Wait_Seconds_with_display.vi"("Message"="Please rotate the probe you are calibrating", "Seconds to wait"=10000.0) -> ()  [unwired: 2 out]
              }
            }
            n223 = local read "Establishment time"() -> (w572:string)
            n224 = Bundle By Name(cluster=w573, "Tunnel Speed"=w563) -> (w574:T5)
          }
          frame "Traverse Position" {
            n225 = Index Array(array=w592, index=0 ("Index")) -> (element=w591:dbl)
            n226 = Index Array(array=w592, index=1 ("Index")) -> (element=w590:dbl)
            n227 = Index Array(array=w592, index=2 ("Index")) -> (element=w589:dbl)
            n228 = local read "Establishment time"() -> (w586:string)
            n229 = Bundle By Name(cluster=w588, "Start X"=w591, "Start Y"=w590, "Start Z"=w589) -> (w587:T5)
          }
          frame "Concentration" {
            w597 = nan ("Start X")
            n230 = local read "Wait factor"() -> (w602:dbl)
            n231 = Index Array(array=w609, index=0 ("Index")) -> (element=w600:dbl)
            n232 = case shown="1, Default" w599 {
              tunnel: [w611 w619 100.0] -> w601
              tunnel: w602 -> [w617 w620 _]
              frame 1, Default {
                n233 = local read "Time FFID valve moved"() -> (w614:dbl)
                n234 = Get Date/Time In Seconds() -> (seconds since 1Jan1904=w616:timestamp)
                n235 = Multiply(x=w617, y=35.0) -> (x*y=w613:dbl)
                n236 = To Double Precision Float(number=w616) -> (double precision float=w615:dbl)
                n237 = Subtract(x=w615, y=w614) -> (x-y=w612:dbl)
                n238 = Subtract(x=w613, y=w612) -> (x-y=w611:dbl)
              }
              frame 2 {
                n239 = Multiply(x=w620, y=25.0) -> (x*y=w619:dbl)
              }
              frame 3 {
              }
            }
            n240 = case shown="\"Check VI only\"" w607 {
              tunnel: w600 -> [w624 w625]
              tunnel: [w623 w626] -> w608
              frame "Check VI only" {
                n241 = To Long Integer(number=w624) -> (32bit integer=w623:i32)
              }
              frame "Run VI" {
                n242 = call "Fast_FID_Valve_Control.vi"("Requested Position"=w625) -> ("Achieved Posn."=w626:T22)  [unwired: 6 out]
              }
            }
            n243 = Number To Decimal String(number=w601) -> (decimal integer string=w604:string)  [unwired: 1 out]
            n244 = Concatenate Strings("!Establish Exp Conditions (s) = " ("Message"), w604) -> (w603:string)
            n245 = To Double Precision Float(number=w608) -> (double precision float=→"Valve position":dbl)
            n246 = Bundle By Name(cluster=w598, "Start X"=w597, "Start Y"=w597, "Start Z"=w597) -> (w596:T5)
          }
        }
        n247 = call "Add_Extra_Command.vi"("Traverse line"=w541, "Extra Command"=w539) -> ("Traverse line Out"=w540:T5)
        n248 = call "Set_Measurement_Conditions.vi"("Simulate/Run"=w555, "Currently on Point"=1, "Traverse line"=w540) -> ("Status Cluster"=w545:T21)  [unwired: 2 out]
        n249 = Unbundle By Name(w545) -> ("Status"=w544:T2)
        "Status" <- w544
        n250 = Equal?(x=w544, y=Multi_Run_Status."Continue" ("Status")) -> (x = y?=w551:bool)
        n251 = Equal?(x=User_Specific_mode."Run VI" ("Mode"), y=w555) -> (x = y?=w552:bool)
        n252 = Increment(x=w542) -> (x+1=w549:T1)
        n253 = And(x=w551, y=w552) -> (x .and. y?=w550:bool)
        n254 = Select(t=w542, s=w550, f=w549) -> (s? t:f=w548:T1)
      }
      frame "Measure Calibration Point" {
        n255 = case shown="\"Tunnel Speed\", Default" w633 {
          tunnel: w632 -> [_ w642]
          tunnel: [w636 w641] -> w628
          tunnel: [w634 w640] -> w627
          frame "Tunnel Speed", Default {
            n256 = local read "New Calib Filenames"() -> (w637:path[])
            n257 = Index Array(array=w637, index=0 ("Index")) -> (element=w638:path)
            n258 = call "Calibration.vi"("Mode"=Calib_mode."Take a New Calibration Point", "Calib file"=w638) -> ("Coefficients"=w634:dbl[][], "Status Out"=w636:T2)  [unwired: 1 in, 15 out]
          }
          frame "Concentration" {
            # "St Dev"
            # "Mean"
            n259 = stacked-sequence {
              seq-local: [_ w646 _] -> [_ _ w691]
              seq-local: [_ w645 _] -> [_ _ w690]
              tunnel: w642 -> [_ w649 _]
              tunnel: [_ w647 _] -> w641
              tunnel: [_ _ w692] -> w640
              frame #0 {
                n260 = global write "Meas_global.vi" "Remote control"(TRUE ("Remote control")) -> ()
                n261 = global write "Meas_global.vi" "Raw data option"(enum16{"Save raw data", "Raw data not saved"}."Save raw data" ("Raw data option")) -> ()
              }
              frame #1 {
                n262 = local read "New Calib Filenames"() -> (w650:path[])
                n263 = Index Array(array=w650, index=0 ("Index")) -> (element=w648:path)
                n264 = while {
                  tunnel: [w658] -> w647
                  tunnel: w648 -> [w657]
                  tunnel: w649 -> [w655]
                  tunnel: [w654] -> w646
                  tunnel: [w653] -> w645
                  i -> [w652]
                  stop <- w656 continue-if-true
                  n265 = stacked-sequence {
                    seq-local: [_ w660 _ _] -> [_ _ _ w684]
                    seq-local: [_ _ w669 _] -> [_ _ _ w688]
                    tunnel: [_ w660 _ _] -> w658
                    tunnel: w657 -> [_ w665 _ _]
                    tunnel: [_ _ _ w679] -> w656
                    tunnel: w655 -> [_ w661 _ _]
                    tunnel: [_ _ w670 _] -> w654
                    tunnel: [_ _ w669 _] -> w653
                    tunnel: w652 -> [_ _ _ w686]
                    frame #0 {
                      n266 = global write "Meas_global.vi" "Remote control"(TRUE ("Remote control")) -> ()
                    }
                    frame #1 {
                      n267 = call "Get_Data_Base_file_code.vi"("Results Filename"=w665, "Data Type"="Raw_Calibrations") -> ("Raw Data File Name"=w662:path)  [unwired: 3 out]
                      n268 = call "Measurement.vi"("setup"=Setup."Run Program", "Post Process"=Post_Process."Take New Data", "File"=Save_Data."Save No Data", "Raw data file"=w662, "Setup filename"=w661) -> ("Status Out"=w660:T2)  [unwired: 2 in, 12 out]
                    }
                    frame #2 {
                      n269 = local read "FF Indexes"() -> (w671:i16[])
                      n270 = global read "Meas_global.vi" "Time Trace"() -> (w668:T23[])
                      n271 = for {
                        tunnel: w671 -> [w678] mode=indexing
                        tunnel: [w677] -> w670 mode=indexing
                        tunnel: [w676] -> w669 mode=indexing
                        tunnel: w668 -> [w674]
                        n272 = Index Array(array=w674, index=w678) -> (element=w673:T23)
                        n273 = Unbundle By Name(w673) -> ("Eng Values"=w672:dbl[])
                        n274 = call "De-spiked_Stats.vi"("Raw Signal"=w672, "No of st dev to chop at"=6.0) -> ("mean"=w677:dbl, "standard deviation"=w676:dbl)  [unwired: 1 out]
                      }
                    }
                    frame #3 {
                      n275 = Greater?(x=w688, y=0.15) -> (0:w687:bool[])
                      n276 = Or Array Elements(Boolean array=w687) -> (logical OR=w681:bool)
                      n277 = Less?(x=w686, y=2) -> (x < y?=w682:bool)
                      n278 = Equal?(x=w684, y=Multi_Run_Status."Continue" ("Status Out")) -> (x = y?=w680:bool)
                      n279 = Compound Arithmetic op=AND(w680, w681, w682) -> (w679:bool)
                    }
                  }
                }
              }
              frame #2 {
                n280 = local read "FFID St Dev"() -> (w695:dbl[][])
                n281 = local read "Valve position"() -> (w699:dbl)
                n282 = local read "Concentrations"() -> (w693:dbl[])
                n283 = global read "Meas_global.vi" "Temp"() -> (w700:dbl)
                n284 = Build Array (concatenate)(w691, w690) -> (w694:dbl[])
                n285 = Build Array (concatenate)(w695, w694) -> (→"FFID St Dev":dbl[][])
                n286 = Index Array(array=w693, index=w699) -> (element=w698:dbl)
                n287 = local read "New Calib Filenames"() -> (w697:path[])
                n288 = for {
                  tunnel: w691 -> [w706] mode=indexing
                  tunnel: w700 -> [w705]
                  tunnel: w698 -> [w704]
                  tunnel: [w703] -> w692 mode=indexing
                  tunnel: w697 -> [w702] mode=indexing
                  tunnel: w690 -> [w701] mode=indexing
                  n289 = stacked-sequence {
                    tunnel: w706 -> [w712 _]
                    tunnel: w705 -> [w709 _]
                    tunnel: w704 -> [w711 _]
                    tunnel: [_ w714] -> w703
                    tunnel: w702 -> [_ w713]
                    tunnel: w701 -> [w707 _]
                    frame #0 {
                      n290 = Build Array(w711, w712, w707, 0.0 ("element"), w709) -> (w710:dbl[])
                      n291 = global write "Calib_global.vi" "Calibration Points"(w710) -> ()
                    }
                    frame #1 {
                      n292 = call "Calibration.vi"("Mode"=Calib_mode."Refit Curve", "Calib file"=w713) -> ("Coefficients"=w715:dbl[][])  [unwired: 1 in, 16 out]
                      n293 = Index Array(array=w715, index (row)=0 ("Index")) -> (element=w714:dbl[])  [unwired: 1 in]
                    }
                  }
                }
              }
            }
          }
        }
        "Coefficients" <- w627
        n294 = local write "Status"(w628) -> ()
      }
      frame "Do Another Calibration Point?" {
        n295 = local read "No of Calib Points"() -> (w731:i32)
        n296 = local read "Status"() -> (w727:T2)
        n297 = local read "Currently On"() -> (w723:i32)
        n298 = case shown="\"Terminate Run\"" w727 {
          tunnel: [w741 w742 TRUE w745] -> w729
          tunnel: [w741 w742 FALSE w745] -> w730
          frame "Continue", Default {
            w741 = TRUE
          }
          frame "Jump to Next Point" {
            w742 = TRUE
          }
          frame "Jump to Next Row" {
          }
          frame "Terminate Run" {
            w745 = FALSE
          }
        }
        n299 = Greater?(x=w731, y=w723) -> (0:w728:bool)
        n300 = Compound Arithmetic op=AND(invert "stop", w729) -> (w726:bool)
        n301 = Compound Arithmetic op=AND(w726, w730, w728) -> (w724:bool)
        n302 = case shown="False" w724 {
          tunnel: w723 -> [_ w740]
          tunnel: [w734 Auto_Calib_Case."Set Measurement Conditions" ("Currently in Case")] -> w722
          tunnel: w721 -> [w735 _]
          tunnel: w720 -> [w733 _]
          frame False {
            n303 = case shown="\"Check VI only\"" w735 {
              tunnel: [Auto_Calib_Case."End" ("Currently in Case") Auto_Calib_Case."Skip Next Frame?" ("Currently in Case")] -> w734
              tunnel: w733 -> [_ _]
              frame "Check VI only" {
              }
              frame "Run VI" {
              }
            }
          }
          frame True {
            n304 = Increment(x=w740) -> (x+1=w739:i32)
            n305 = local write "Currently On"(w739) -> ()
          }
        }
        n306 = case shown="True" "stop" {
          frame False {
          }
          frame True {
            n307 = local write "Status"(Multi_Run_Status."Terminate Run" ("Status")) -> ()
          }
        }
      }
      frame "Skip Next Frame?" {
        n308 = local read "Status"() -> (w749:T2)
        n309 = case shown="\"Tunnel Speed\", Default" w746 {
          frame "Tunnel Speed", Default {
          }
          frame "Concentration" {
            n310 = call "Fast_FID_Valve_Control.vi"("Requested Position"=4 ("Requested Posn.")) -> ()  [unwired: 7 out]
          }
        }
        n311 = case shown="\"Continue\"" w749 {
          tunnel: [w753 Auto_Calib_Case."End" ("Currently in Case")] -> w748
          tunnel: w747 -> [w753 _]
          frame "Continue" {
          }
          frame "Terminate Run", Default {
          }
        }
      }
      frame "Insert New calibration Filenames into Measurement Setup file" {
        n312 = local read "New Calib Filenames"() -> (w755:path[])
        n313 = global read "Meas_global.vi" "Raw data file"() -> (w765:path)
        n314 = local read "Ch No's"() -> (w756:i16[])
        n315 = Strip Path(path=w765) -> (stripped path=w764:path)  [unwired: 1 out]
        n316 = Equal?(x=Auto_Calib_Type."Concentration" ("Calibration varying"), y=w762) -> (x = y?=w761:bool)
        n317 = call "Current_Calib_Filenames.vi"("Calib Filename"=w755, "Channel Numbers"=w756, "Mode"=App_Global."Write to Global") -> ()  [unwired: 3 out]
        n318 = case shown="False" w761 {
          tunnel: [Auto_Calib_Case."Warn if Current Calibration fit is poor" ("Currently in Case") w772] -> w760
          tunnel: w759 -> [_ w772]
          tunnel: w755 -> [_ w771]
          tunnel: [1 w770] -> w758
          frame False {
          }
          frame True {
            n319 = Array Size(array=w771) -> (size(s)=w770:i32)
          }
        }
        n320 = for {
          N: w758 -> [_]
          tunnel: w755 -> [w774] mode=indexing
          tunnel: w764 -> [w778]
          w776 = FALSE  # Variable Target?
          n321 = Strip Path(path=w774) -> (name=w777:string)  [unwired: 1 out]
          n322 = Build Path(base path=w778, name or relative path=w777) -> (appended path=w773:path)
          n323 = call "Remember_Calib_Filenames.vi"("Filename to Remember"=w773) -> ()  [unwired: 1 out]
          n324 = call "Copy_with_Check.vi"("Mode"=enum16{"Move", "Copy"}."Copy", "Target Path"=w773, "Variable Target?"=w776, "Source Path"=w774) -> ()  [unwired: 1 out]
        }
      }
      frame "Warn if FFID calibration is very non linear" {
        w795 = FALSE  # Dialog Box (T)
        n325 = local read "Root Name"() -> (w794:string[])
        n326 = local read "Coefficients"() -> (w797:dbl[][])
        n327 = for {
          tunnel: w797 -> [w804] mode=indexing
          shift-right: [w806] -> w792
          shift-left: "" -> [w807]
          tunnel: w794 -> [w808] mode=indexing
          tunnel: [w801] -> w787 mode=indexing
          tunnel: "If the calibration fit for %s had been linear instead of a second order polynomial, it would have yielded an average fit error of %.1f%%.\\n" ("Format String") -> [w799]
          n328 = Index Array(array=w804, index=0 ("Index")) -> (element=w802:dbl)
          n329 = Absolute Value(x=w802) -> (abs(x)=w801:dbl)
          n330 = Less?(x=w801, y=2.2) -> (x < y?=w805:bool)
          n331 = case shown="False" w805 {
            tunnel: w808 -> [w810 _]
            tunnel: w801 -> [w811 _]
            tunnel: w807 -> [w814 w815]
            tunnel: [w812 w815] -> w806
            tunnel: w799 -> [w809 _]
            frame False {
              n332 = Format Into String(format string=w809, w810, w811) -> (resulting string=w813:string)  [unwired: 2 in, 1 out]
              n333 = Concatenate Strings(w814, w813) -> (w812:string)
            }
            frame True {
            }
          }
        }
        n334 = Array Max & Min(array=w787) -> (max value=w786:dbl)  [unwired: 3 out]
        n335 = Greater?(x=w786, y=7.0) -> (0:w784:bool)
        n336 = Select(t="Very Poor FFID Linearity", s=w784, f="Poor FFID Linearity") -> (s? t:f=w781:string)
        n337 = Empty String/Path?(string/path=w792) -> (empty?=w791:bool)
        n338 = Not(x=w791) -> (.not. x?=w790:bool)
        n339 = Bundle By Name(cluster=errorcluster {"status"=FALSE, "code"=0, "source"=""} ("error in (no error)"), "source"=w792, "status"=w790) -> (w789:errorcluster)
        n340 = call "EnFlo_Error_Handler.vi"("error in (no error)"=w789, "Error Type"=w781, "Dialog Box (T)"=w795) -> ()  [unwired: 3 out]
      }
      frame "Warn if FFID variance is high" {
        w837 = FALSE  # Dialog Box (T)
        n341 = local read "New Calib Filenames"() -> (w819:path[])
        n342 = local read "FFID St Dev"() -> (w839:dbl[][])
        n343 = Index Array(array=w824, index (col)=0 ("disabled index (col)")) -> (element=w822:dbl[])  [unwired: 1 in]
        n344 = Array Size(array=w819) -> (size(s)=w818:i32)
        n345 = for {
          tunnel: w839 -> [w856]
          shift-right: [w858] -> w835
          shift-left: "" -> [w859]
          tunnel: w819 -> [w847] mode=indexing
          tunnel: "For %s the measurement at %dppm had a standard deviation of %.2f volts for an average value of  %.1f volts.\\n" ("Format String") -> [w857]
          tunnel: w822 -> [w850]
          tunnel: [w849] -> w820 mode=indexing
          tunnel: w818 -> [w845]
          tunnel: [w841] -> w816 mode=indexing
          i -> [w844]
          n346 = Add(x=w845, y=w844) -> (x+y=w843:i32)
          n347 = Strip Path(path=w847) -> (name=w846:string)  [unwired: 1 out]
          n348 = Index Array(array=w856, index (col)=w844) -> (element=w848:dbl[])  [unwired: 1 in]
          n349 = Index Array(array=w856, index (col)=w843) -> (element=w842:dbl[])  [unwired: 1 in]
          n350 = Array Max & Min(array=w842) -> (min value=w841:dbl)  [unwired: 3 out]
          n351 = call-poly <vilib>:"Mean.vi"("X"=w848) -> ("mean"=w855:dbl)  [unwired: 1 out]
          n352 = Divide(x=w842, y=w855) -> (x/y=w854:dbl[])
          n353 = Array Max & Min(array=w854) -> (max value=w849:dbl, max index (indices)=w851:i32)  [unwired: 2 out]
          n354 = Greater?(x=w849, y=0.06) -> (0:w852:bool)
          n355 = case shown="True" w852 {
            tunnel: w846 -> [_ w870]
            tunnel: w859 -> [w860 w876]
            tunnel: [w860 w874] -> w858
            tunnel: w857 -> [_ w873]
            tunnel: w851 -> [_ w871]
            tunnel: w850 -> [_ w872]
            tunnel: w849 -> [_ _]
            tunnel: w842 -> [_ w869]
            tunnel: w848 -> [_ w867]
            frame False {
            }
            frame True {
              n356 = local read "Concentrations"() -> (w865:dbl[])
              n357 = Index Array(array=w872, index=w871) -> (element=w866:dbl)
              n358 = Index Array(array=w869, index=w871) -> (element=w863:dbl)
              n359 = Index Array(array=w867, index=w871) -> (element=w868:dbl)
              n360 = Index Array(array=w865, index=w866) -> (element=w864:dbl)
              n361 = Multiply(x=w863, y=2.5) -> (x*y=w862:dbl)
              n362 = Format Into String(format string=w873, w870, w864, w862, w868) -> (resulting string=w875:string)  [unwired: 2 in, 1 out]
              n363 = Concatenate Strings(w876, w875) -> (w874:string)
            }
          }
        }
        "Minimum St Dev" <- w816
        n364 = Array Max & Min(array=w820) -> (max value=w830:dbl)  [unwired: 3 out]
        n365 = Greater?(x=w830, y=0.09) -> (0:w828:bool)
        n366 = Select(t="Very unstable FFID calibration point", s=w828, f="Unstable FFID calibration point") -> (s? t:f=w825:string)
        n367 = Empty String/Path?(string/path=w835) -> (empty?=w834:bool)
        n368 = Not(x=w834) -> (.not. x?=w833:bool)
        n369 = Bundle By Name(cluster=errorcluster {"status"=FALSE, "code"=0, "source"=""} ("error in (no error)"), "source"=w835, "status"=w833) -> (w832:errorcluster)
        n370 = call "EnFlo_Error_Handler.vi"("error in (no error)"=w832, "Error Type"=w825, "Dialog Box (T)"=w837) -> ()  [unwired: 3 out]
      }
      frame "Insert Bkgnd Variance into calib file" {
        n371 = local read "New Calib Filenames"() -> (w879:path[])
        n372 = local read "Minimum St Dev"() -> (w880:dbl[])
        n373 = local read "Coefficients"() -> (w877:dbl[][])
        n374 = for {
          tunnel: w880 -> [w885] mode=indexing
          tunnel: w879 -> [w891] mode=indexing
          tunnel: w877 -> [w888] mode=indexing
          n375 = call "Read_File_Simple.vi"("Filename"=w891) -> ("string"=w895:string)  [unwired: 2 in, 7 out]
          n376 = Index Array(array=w888, index=2) -> (element=w886:dbl)
          n377 = Multiply(x=w885, y=w886) -> (x*y=w884:dbl)
          n378 = Square(x=w884) -> (x^2=w883:dbl)
          n379 = Number To Fractional String(number=w883, precision (6)=i16 8) -> (F-format string=w893:string)  [unwired: 2 out]
          n380 = call "Replace_data_in_setup_string.vi"("New data string"=w893, "Input string"=w895, "Variable name"="Fast FID Bkgnd Variance") -> ("Appended string"=w890:string)
          n381 = call "Write_File_Simple.vi"("append to file? (new file:F)"=FALSE, "character string"=w890, "file path"=w891) -> ()  [unwired: 2 out]
        }
      }
      frame "Warn if FFID voltages are too low" {
        w913 = FALSE  # Dialog Box (T)
        n382 = local read "Coefficients"() -> (w903:dbl[][])
        n383 = local read "Concentrations"() -> (w899:dbl[])
        n384 = Index Array(array=w906, index (col)=0 ("disabled index (col)")) -> (element=w898:dbl[])  [unwired: 1 in]
        n385 = local read "New Calib Filenames"() -> (w902:path[])
        n386 = for {
          tunnel: w899 -> [w918]
          tunnel: w898 -> [w917] mode=indexing
          tunnel: [w916] -> w897 mode=indexing
          n387 = Index Array(array=w918, index=w917) -> (element=w916:dbl)
        }
        n388 = Array Max & Min(array=w897) -> (max value=w896:dbl)  [unwired: 3 out]
        n389 = for {
          shift-right: [w928] -> w911
          shift-left: "" -> [w929]
          tunnel: "For %s the maximum measured calibration voltage was %.1f volts.\nCheck that the FID is running and correctly connected to the acquisition system." ("Format String") -> [w927]
          tunnel: w903 -> [w925] mode=indexing
          tunnel: w902 -> [w921] mode=indexing
          tunnel: w896 -> [w920]
          n390 = Split 1D Array(array=w925, index=1) -> (second subarray=w924:dbl[])  [unwired: 1 out]
          n391 = call "Polybackwards.vi"("Coefficients"=w924, "Y input"=w920) -> ("X output"=w919:dbl)  [unwired: 1 out]
          n392 = Less?(x=w919, y=0.2) -> (x < y?=w922:bool)
          n393 = case shown="True" w922 {
            tunnel: w929 -> [w930 w937]
            tunnel: [w930 w935] -> w928
            tunnel: w927 -> [_ w934]
            tunnel: w921 -> [_ w933]
            tunnel: w919 -> [_ w931]
            frame False {
            }
            frame True {
              n394 = Strip Path(path=w933) -> (name=w932:string)  [unwired: 1 out]
              n395 = Format Into String(format string=w934, w932, w931) -> (resulting string=w936:string)  [unwired: 2 in, 1 out]
              n396 = Concatenate Strings(w937, w936) -> (w935:string)
            }
          }
        }
        n397 = Empty String/Path?(string/path=w911) -> (empty?=w910:bool)
        n398 = Not(x=w910) -> (.not. x?=w909:bool)
        n399 = Bundle By Name(cluster=errorcluster {"status"=FALSE, "code"=0, "source"=""} ("error in (no error)"), "source"=w911, "status"=w909) -> (w908:errorcluster)
        n400 = call "EnFlo_Error_Handler.vi"("error in (no error)"=w908, "Error Type"="Low FFID calibration voltages", "Dialog Box (T)"=w913) -> ()  [unwired: 3 out]
      }
      frame "Warn if Current Calibration fit is poor" {
        w952 = FALSE  # Dialog Box (T)
        n401 = local read "Root Name"() -> (w951:string[])
        n402 = local read "Coefficients"() -> (w954:dbl[][])
        n403 = for {
          tunnel: w954 -> [w961] mode=indexing
          shift-right: [w963] -> w949
          shift-left: "" -> [w964]
          tunnel: w951 -> [w965] mode=indexing
          tunnel: [w958] -> w944 mode=indexing
          n404 = Index Array(array=w961, index=0 ("Index")) -> (element=w959:dbl)
          n405 = Absolute Value(x=w959) -> (abs(x)=w958:dbl)
          n406 = Less?(x=w958, y=1.0) -> (x < y?=w962:bool)
          n407 = case shown="True" w962 {
            tunnel: w965 -> [w967 _]
            tunnel: w958 -> [w968 _]
            tunnel: w964 -> [w971 w972]
            tunnel: [w969 w972] -> w963
            frame False {
              n408 = Format Into String(format string="The calibration for %s has an average fit error of %.1f%%\\n" ("Format String"), w967, w968) -> (resulting string=w970:string)  [unwired: 2 in, 1 out]
              n409 = Concatenate Strings(w971, w970) -> (w969:string)
            }
            frame True {
            }
          }
        }
        n410 = Array Max & Min(array=w944) -> (max value=w943:dbl)  [unwired: 3 out]
        n411 = Greater?(x=w943, y=7.0) -> (0:w941:bool)
        n412 = Select(t="Very Poor Calibration", s=w941, f="Poor Calibration") -> (s? t:f=w938:string)
        n413 = Empty String/Path?(string/path=w949) -> (empty?=w948:bool)
        n414 = Not(x=w948) -> (.not. x?=w947:bool)
        n415 = Bundle By Name(cluster=errorcluster {"status"=FALSE, "code"=0, "source"=""} ("error in (no error)"), "source"=w949, "status"=w947) -> (w946:errorcluster)
        n416 = call "EnFlo_Error_Handler.vi"("error in (no error)"=w946, "Error Type"=w938, "Dialog Box (T)"=w952) -> ()  [unwired: 3 out]
      }
      frame "Warn if Calibration Coefficients have significantly altered" {
        w998 = FALSE  # Dialog Box (T)
        w985 = 8.0 ("y")
        n417 = local read "New Calib Filenames"() -> (w990:path[])
        n418 = local read "Root Name"() -> (w989:string[])
        n419 = global read "Calib_global.vi" "Instrument type"() -> (w988:T14)
        n420 = Unbundle By Name(w977) -> ("Extra Commands"=w976:string)
        n421 = global read "Extra_Commands_Global.vi" "If Command"() -> (w978:string)
        n422 = call "Extra_Commands.vi"("String to Search"=w976, "Command"=w978) -> ("String Value"=w975:string)  [unwired: 1 in, 4 out]
        n423 = call "Calibration_Analysis.vi"("Root Name"=w989, "New Calib Filenames"=w990, "Instrument type"=w988, "Clear Calib History"="Clear Calib History") -> ("Error String"=w987:string, "Max % Error"=w973:dbl)
        n424 = call "Get_array_values_fr_String.vi"("String Value"=w975) -> ("Numeric Array"=w974:dbl[], "String array"=w980:string[])
        n425 = Greater?(x=w973, y=w985) -> (0:w986:bool)
        n426 = Index Array(array=w980, index=0 ("Index")) -> (element=w981:string)
        n427 = case shown="\"Drift Greater Than\"" w981 {
          tunnel: w974 -> [w1004 _]
          tunnel: w973 -> [w1003 _]
          frame "Drift Greater Than" {
            n428 = Index Array(array=w1004, index=1 ("Index")) -> (element=w1002:dbl)
            n429 = Greater?(x=w1003, y=w1002) -> (0:w1001:bool)
            n430 = case shown="True" w1001 {
              frame False {
              }
              frame True {
                n431 = local write "Status"(Multi_Run_Status."Jump To Fall Back" ("Status")) -> ()
              }
            }
          }
          frame "No Match", Default {
          }
        }
        n432 = Format Into String(format string="Calibration Drift Greater than %d%%", w985) -> (resulting string=w983:string)  [unwired: 2 in, 1 out]
        n433 = Select(t=w983, s=w986, f="Calibration Drift") -> (s? t:f=w991:string)
        n434 = Empty String/Path?(string/path=w987) -> (empty?=w996:bool)
        n435 = Not(x=w996) -> (.not. x?=w995:bool)
        n436 = Bundle By Name(cluster=errorcluster {"status"=FALSE, "code"=0, "source"=""} ("error in (no error)"), "source"=w987, "status"=w995) -> (w994:errorcluster)
        n437 = call "EnFlo_Error_Handler.vi"("error in (no error)"=w994, "Error Type"=w991, "Dialog Box (T)"=w998) -> ()  [unwired: 3 out]
      }
      frame "End" {
        n438 = case shown="\"Concentration\"" w1010 {
          tunnel: w1008 -> [_ w1027]
          tunnel: w1009 -> [_ w1015]
          tunnel: w1007 -> [_ w1026]
          frame "Tunnel Speed", Default {
          }
          frame "Concentration" {
            n439 = Unbundle By Name(w1027) -> ("Averaging time (min)"=w1029:dbl)
            n440 = global read "Trav_pos_global.vi" "Simulation Time"() -> (w1018:timestamp)
            n441 = Unbundle By Name(w1027) -> ("Start Z"=w1014:dbl)
            n442 = Select(t=3 ("No. of pts."), s=w1026, f=2 ("No. of pts.")) -> (s? t:f=w1020:i32)
            n443 = Multiply(x=60.0, y=w1029) -> (x*y=w1023:dbl)
            n444 = Add(x=w1014, y=50.0) -> (x+y=w1030:dbl)
            n445 = Add(x=w1023, y=60.0) -> (x+y=w1021:dbl)
            n446 = Bundle By Name(cluster=w1027, "Start Z"=w1030) -> (w1031:T5)
            n447 = Multiply(x=w1021, y=w1020) -> (x*y=w1019:dbl)
            n448 = Add(x=w1018, y=w1019) -> (x+y=w1016:timestamp)
            n449 = call "Set_Traverse_Position.vi"("Simulate/Run"=w1015, "Currently on Point"=1, "Traverse line"=w1031) -> ()  [unwired: 3 out]
            n450 = call "Run_FFID_Bkgnd.vi"("Simulated Time"=w1016, "Run Now?"=TRUE, "Simulate/Run"=w1015) -> ()  [unwired: 3 out]
          }
        }
        "Traverse Out" <- w1008
      }
    }
    "Currently in Case" <- w16
  }
  "Error Messages" <- w10
